vi "PrimaryInterfaceGetVariableValue.vi"(8 "Variable":refnum<k24>, 11 "error in":errorcluster) -> (0 "Value":T1, 3 "error out":errorcluster)   [LabVIEW 2022 SP3, in "UnderAutomation.UniversalRobots.lvlib"]
uses:
  UnderAutomation.UniversalRobots.lvlib
  C:/Users/fg/Documents/UniversalRobots.vi/LabVIEW_2024/UnderAutomation.UniversalRobots/lib/UnderAutomation.UniversalRobots.dll
  LabVIEW_2024/UnderAutomation.UniversalRobots/lib/UnderAutomation.UniversalRobots.dll
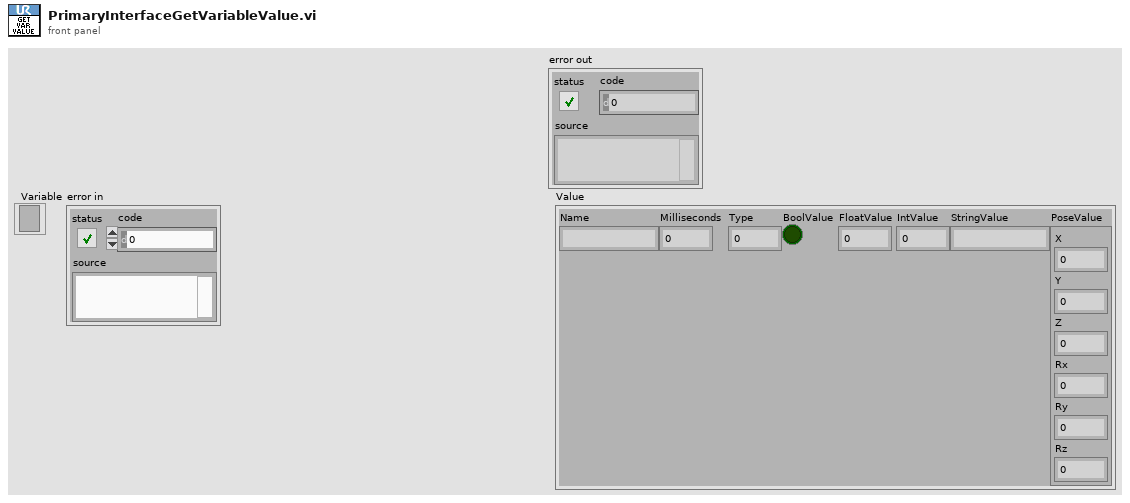
[diagram p1: front panel]
types:
  T1 = cluster{"Name":string, "Milliseconds":i32, "Type":i32, "BoolValue":bool, "FloatValue":sgl, "IntValue":i32, "StringValue":string, "PoseValue":cluster{"X":dbl, "Y":dbl, "Z":dbl, "Rx":dbl, "Ry":dbl, "Rz":dbl}}
  T2 = cluster{"X":dbl, "Y":dbl, "Z":dbl, "Rx":dbl, "Ry":dbl, "Rz":dbl}
  T3 = cluster{"Name":string, "Milliseconds":i32, "Type":i32, "ToBool":bool, "ToFloat":sgl, "ToInt":i32, "ToString":string, cluster{"X":dbl, "Y":dbl, "Z":dbl, "Rx":dbl, "Ry":dbl, "Rz":dbl}}
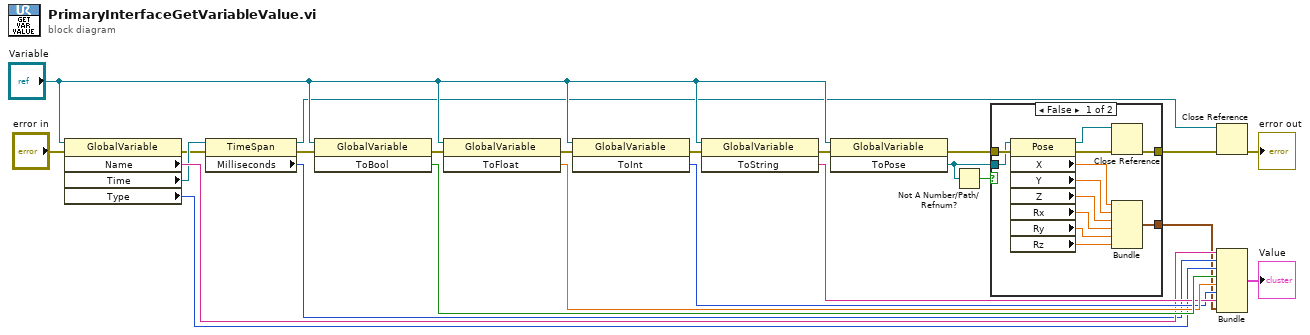
[diagram p0: block diagram]
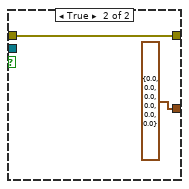
[diagram p2: hidden frame]
diagram:
  n1 = property class="GlobalVariable"(reference="Variable", error in="error in") -> (error out=w13:errorcluster, "Name"=w20:string, "Time"=w18:refnum<k24>, "Type"=w19:i32)  [unwired: 1 out]
  n2 = property class="TimeSpan"(reference=w18, error in=w13) -> (reference out=w1:refnum<k24>, error out=w12:errorcluster, "Milliseconds"=w17:i32)
  n3 = invoke class="GlobalVariable" method="ToBool"(reference="Variable", error in=w12) -> (error out=w11:errorcluster, "ToBool"=w24:bool)  [unwired: 1 in, 1 out]
  n4 = invoke class="GlobalVariable" method="ToFloat"(reference="Variable", error in=w11) -> (error out=w10:errorcluster, "ToFloat"=w23:sgl)  [unwired: 1 in, 1 out]
  n5 = invoke class="GlobalVariable" method="ToInt"(reference="Variable", error in=w10) -> (error out=w9:errorcluster, "ToInt"=w21:i32)  [unwired: 1 in, 1 out]
  n6 = invoke class="GlobalVariable" method="ToString"(reference="Variable", error in=w9) -> (error out=w8:errorcluster, "ToString"=w22:string)  [unwired: 1 in, 1 out]
  n7 = invoke class="GlobalVariable" method="ToPose"(reference="Variable", error in=w8) -> (error out=w7:errorcluster, "ToPose"=w4:refnum<k24>)  [unwired: 1 in, 1 out]
  n8 = Not A Number/Path/Refnum?(number/path/refnum=w4) -> (NaN/Path/Refnum?=w5:bool)
  n9 = case shown="False" w5 {
    tunnel: w7 -> [w30 w38]
    tunnel: [w29 T2 {"X"=0.0, "Y"=0.0, "Z"=0.0, "Rx"=0.0, "Ry"=0.0, "Rz"=0.0}] -> w6
    tunnel: [w26 w38] -> w3
    tunnel: w4 -> [w28 _]
    frame False {
      n10 = property class="Pose"(reference=w28, error in=w30) -> (reference out=w25:refnum<k24>, error out=w27:errorcluster, "X"=w31:dbl, "Y"=w32:dbl, "Z"=w33:dbl, "Rx"=w34:dbl, "Ry"=w35:dbl, "Rz"=w36:dbl)
      n11 = Close Reference(reference=w25, error in (no error)=w27) -> (error out=w26:errorcluster)
      n12 = Bundle("X"=w31, "Y"=w32, "Z"=w33, "Rx"=w34, "Ry"=w35, "Rz"=w36) -> (w29:T2)  [unwired: 1 in]
    }
    frame True {
    }
  }
  n13 = Close Reference(reference=w1, error in (no error)=w3) -> (error out=→"error out":errorcluster)
  n14 = Bundle("Name"=w20, "Milliseconds"=w17, "Type"=w19, "ToBool"=w24, "ToFloat"=w23, "ToInt"=w21, "ToString"=w22, w6) -> (→"Value":T3)  [unwired: 1 in]
